vi "_DFH.vi"(0 "System no.":i32=1 min=1 max=4 step=1, 2 "DFH axes":string[](array[string]), 3 "All axes?":bool, 4 "Axis identifier?":bool=TRUE, 5 "error in":errorcluster) -> (19 "error out":errorcluster)   [LabVIEW 2012]
doc: "Defines current position of the \"DFH axes\" as home position. Their position value is set to 0. Due to the change of the home position the values for the travel range limits (TMN?, TMX?) are also changed accordingly. The home position is reset to default by \"ATZ.vi\", \"REF.vi\", \"MNL.vi\", \"MPL.vi\" or similiar command VIs.\n\nValid for C-702, C-843, C-843.PM, C-844, C-848, C-865, C-866, C-880, C-880K005, E-517, E-710, E-755, E-761, Mercury\n\nC-880K005: VI only supported when called through PI_Multix.vi\n\nE-517: If All axes? = TRUE, then Axis identifier? must be TRUE. The values are saved with WPA 100. The position shown in the E-517 display is not affected by DFH because it is that of the sensor channel (can also be queried with TSP?). DFH affects only the axis position which can be queried with POS?.\n\nE-755: If All axes? = TRUE, then Axis identifier? must be TRUE. Command not available for E-755.101.\n\nE-761: If All axes? = TRUE, then Axis identifier? must be TRUE. The values are saved with WPA 100.\n\nAll other systems: If All axes? = TRUE, then Axis identifier? must be TRUE"
panel:
  # "Defines current position of the \"DFH axes\" as home \nposition. Their position value is set to 0. The home\nposition is reset to default by \"ATZ.vi\", \"REF.vi\", \n\"MNL.vi\", \"MPL.vi\" or similiar command VIs."
  # "If all axes: use"
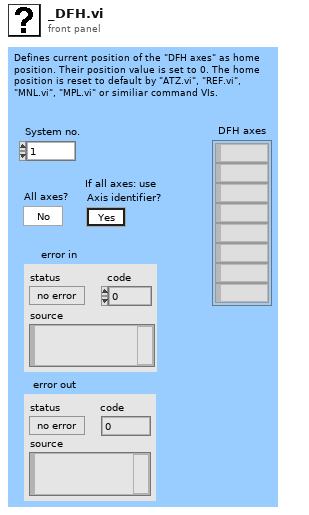
[diagram p1: front panel]
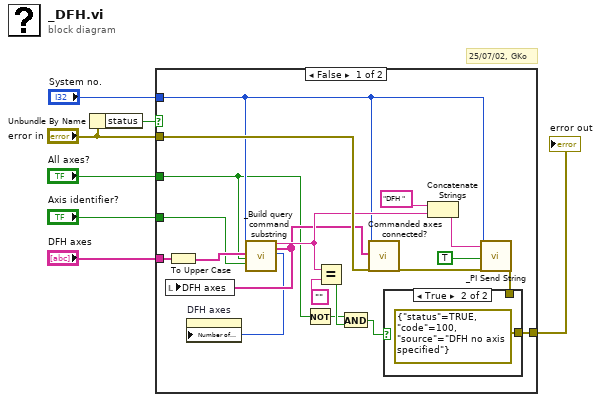
[diagram p0: block diagram]
diagram:
  # "25/07/02, GKo"
  n1 = Unbundle By Name("error in") -> ("status"=w1:bool)
  n2 = case shown="False" w1 {
    tunnel: "error in" -> [w23 w29]
    tunnel: "DFH axes" -> [w22 _]
    tunnel: "Axis identifier?" -> [w19 _]
    tunnel: "System no." -> [w17 _]
    tunnel: "All axes?" -> [w12 _]
    tunnel: [w9 w29] -> w3
    frame False {
      n3 = To Upper Case(1:w22) -> (0:w20:string[])
      n4 = call "_Build query command substring.vi"("System no."=w17, "Axes to query in"=w20, "Query\nAll axes?"=w12, "For all axes: use\nAxis identifier?"=w19) -> ("Command substring"=w18:string, "Axes to query out"=w16:string[], "Number of rows"=w14:u32)  [unwired: 13 in]
      n5 = local write "DFH axes"(w16) -> ()
      n6 = property on="DFH axes" class="Arr (strict)"("Number of Rows"=w14) -> ()  [unwired: 2 in, 2 out]
      n7 = Not(x=w12) -> (.not. x?=w11:bool)
      n8 = Equal?(x=w18, y="" ("x")) -> (x = y?=w13:bool)
      n9 = And(x=w11, y=w13) -> (x .and. y?=w10:bool)
      n10 = call "Commanded axes connected?.vi"("System no."=w17, "Commanded axes"=w16, "error in"=w23) -> ("error out"=w15:errorcluster)  [unwired: 15 in, 1 out]
      n11 = Concatenate Strings("DFH ", w18) -> (w24:string)
      n12 = call "_PI Send String.vi"("System no."=w17, "String to send"=w24, "Attach termination char.?"=TRUE ("Attach Linefeed?"), "error in"=w15) -> ("error out"=w8:errorcluster)  [unwired: 15 in]
      n13 = case shown="True" w10 {
        tunnel: [w27 errorcluster {"status"=TRUE, "code"=100, "source"="DFH no axis specified"} ("error out")] -> w9
        tunnel: w8 -> [w27 _]
        frame False {
        }
        frame True {
        }
      }
    }
    frame True {
    }
  }
  "error out" <- w3
